vi "Main.vi"(11 "Module Admin":refnum<class "Delacor_lib_QMH_Module Admin.lvclass">) -> ()   [LabVIEW 2020, in "DataBase.lvlib"]
doc: "This template is based off of the Queued Message Handler design pattern and the Queued Message Handler project template that ships with LabVIEW.\n\nThe main difference is that the queue is private to this module and communication between modules is performed via Broadcast and Request events.\n\nRequest events are wrapped in public API methods and are handled in the Event Handling Loop (EHL) of this VI. Any module can register for Broadcast events sent by this module. The EHL generates messages based on user interface actions.\n\nThe Message Handling Loop (MHL) processes messages generated by the EHL, or by other messages. The messages are string values, so new messages can be added easily to the Message Cases case structure in the MHL. Each message cluster can also provide an optional value for Message Data, which is a variant that can be converted to whatever message-specific data is required.\n_____\nBased on Delacor QMH Project Template 5.0.0.82."
uses:
  DataBase.lvlib
  <vilib>/Delacor/Delacor QMH/Libraries/Module Admin_class/Delacor_lib_QMH_Module Admin.lvclass
  Module Data--cluster.ctl
  Acquisition/SignalConfig--cluster.ctl
  Stop Argument--cluster.ctl
  <vilib>/Delacor/Delacor QMH/Libraries/Message Queue_class/Delacor_lib_QMH_Message Queue.lvclass/Delacor_lib_QMH_Message Queue.ctl
  <vilib>/Delacor/Delacor QMH/Libraries/Module Admin_class/Delacor_lib_QMH_Module Admin.lvclass/Delacor_lib_QMH_Module Admin.ctl
  Fetch Data Argument--cluster.ctl
  Fetch Data (Reply Payload)--cluster.ctl
  Save Signal Config Argument--cluster.ctl
  Read Config From DB Argument--cluster.ctl
  Read Config From DB (Reply Payload)--cluster.ctl
  <vilib>/Delacor/Delacor QMH/Libraries/Message Queue_class/Delacor_lib_QMH_Enqueue Message (Single).vi
  <vilib>/Delacor/Delacor QMH/Libraries/Module Admin_class/Delacor_lib_QMH_Get External Launch.vi
  <vilib>/Utility/error.llb/Error Cluster From Error Code.vi
  <vilib>/ErrorRing/Error Ring.xnode
  <vilib>/Delacor/Delacor QMH/Libraries/Message Queue_class/Delacor_lib_QMH_Message Queue.lvclass
panel:
  out "error out":errorcluster
  out "Status":string
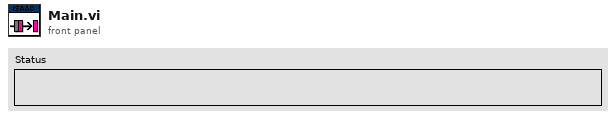
[diagram p1: front panel]
types:
  T1 = typedef "DataBase.lvlib/Request Events--cluster.ctl" = cluster{"Stop Module":refnum<user-event>, "Show Panel":refnum<user-event>, "Hide Panel":refnum<user-event>, "Get Module Execution Status":refnum<user-event>, "Show Diagram":refnum<user-event>, "Fetch Data":refnum<user-event>, "Save config":refnum<user-event>, "Save Signal Config":refnum<user-event>, "Read Config From DB":refnum<user-event>}
  T2 = typedef "DataBase.lvlib/Module Data--cluster.ctl" = cluster{"Status":string, "SignalConfig":T3}
  T3 = typedef "SignalConfig--cluster.ctl" = cluster{"VPP":i32, "Frecuency":dbl, "Offset":dbl, "signal type":enum16{"Sine Wave", "Triangle Wave", "Square Wave", "Sawtooth Wave"}}
  T4 = enum32{"invalid lock state", "Not Locked", "Locked (No Password)", "Password-protected"}
  T5 = typedef "DataBase.lvlib/Stop Argument--cluster.ctl" = cluster{"Origin":string, "Exit via Stop Module Req?":bool, "Wait for Module to stop?":bool}
  T6 = typedef "DataBase.lvlib/Fetch Data Argument--cluster.ctl" = cluster{"End Time":timestamp, "Start Time":timestamp, "Data Results":refnum<vi>, "Wait Notifier":refnum<notifier>, "wait for reply":bool}
  T7 = typedef "DataBase.lvlib/Save Signal Config Argument--cluster.ctl" = cluster{"SignalConfig":T3}
  T8 = typedef "DataBase.lvlib/Read Config From DB Argument--cluster.ctl" = cluster{"Wait Notifier":refnum<notifier>, "wait for reply":bool}
  T9 = enum32{"Invalid", "Standard", "Closed", "Hidden", "Minimized", "Maximized"}
  T10 = typedef "DataBase.lvlib/Fetch Data (Reply Payload)--cluster.ctl" = cluster{"Reply Payload":cluster{"Data":string[][], "Columns":string[], "FetchFrecuencyData_error":errorcluster}}
  T11 = typedef "DataBase.lvlib/Read Config From DB (Reply Payload)--cluster.ctl" = cluster{"SignalConfig":T3, "Read Config From DB_error":errorcluster}
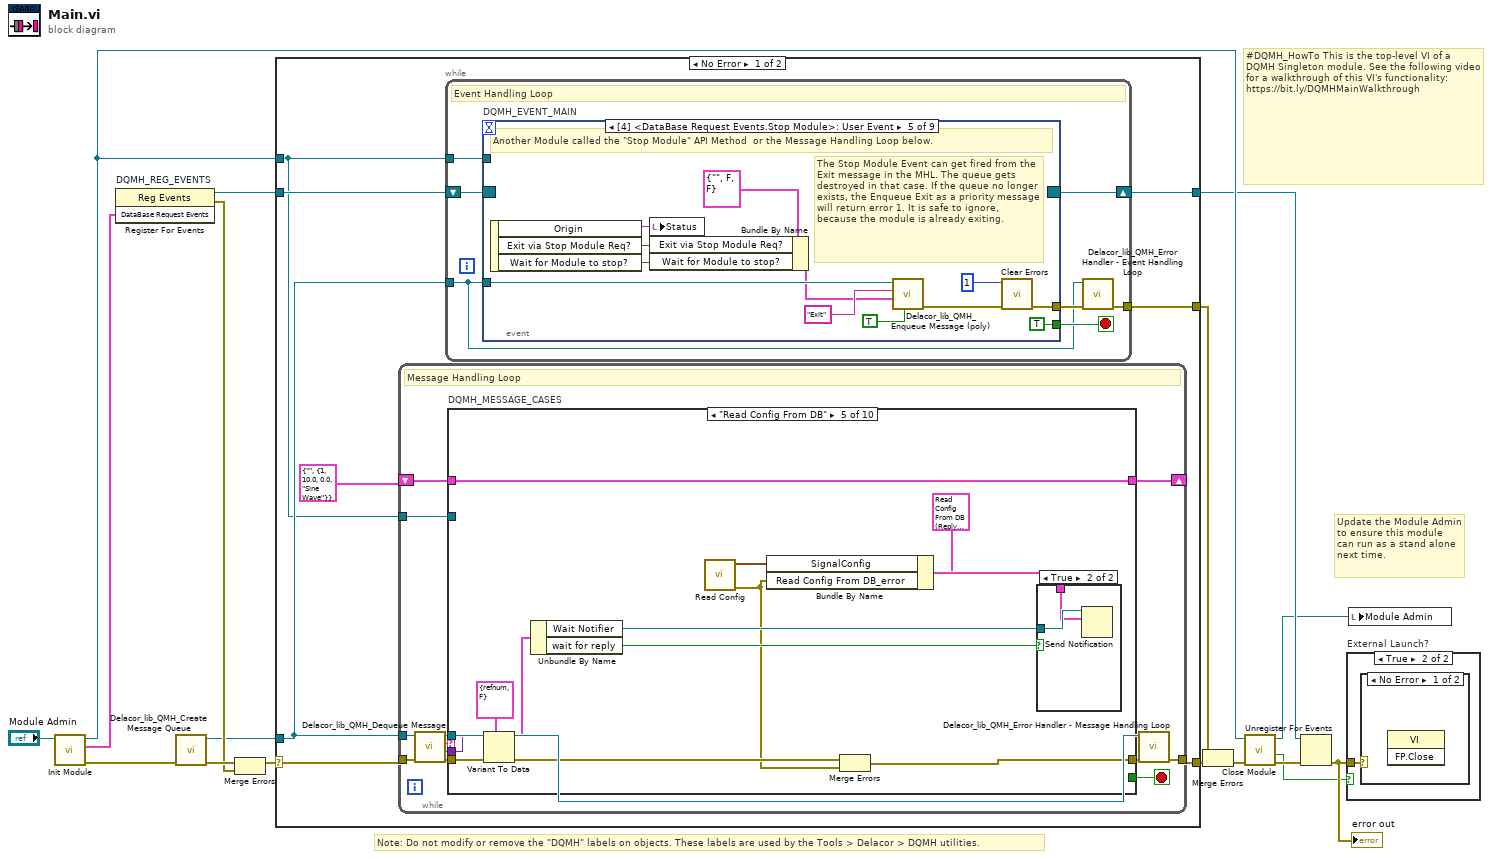
[diagram p0: block diagram]
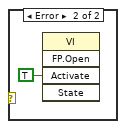
[diagram p3: hidden frame]
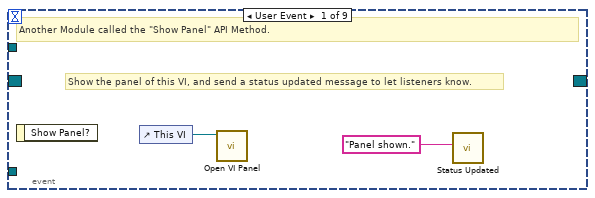
[diagram p4: hidden frame]
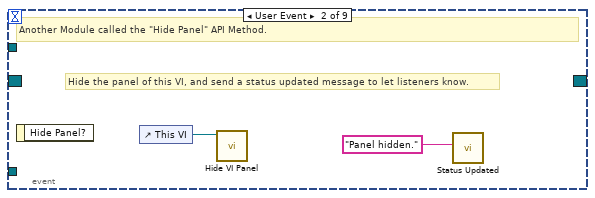
[diagram p5: hidden frame]
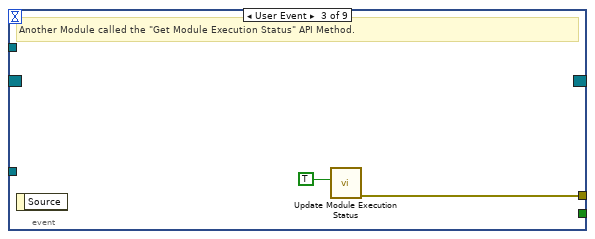
[diagram p6: hidden frame]
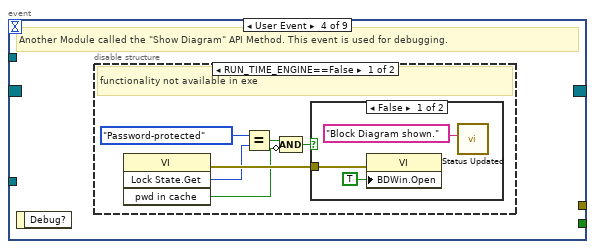
[diagram p7: hidden frame]
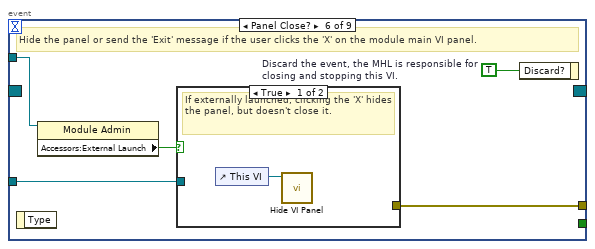
[diagram p10: hidden frame]
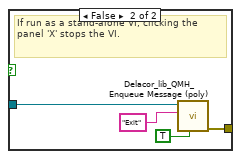
[diagram p11: hidden frame]
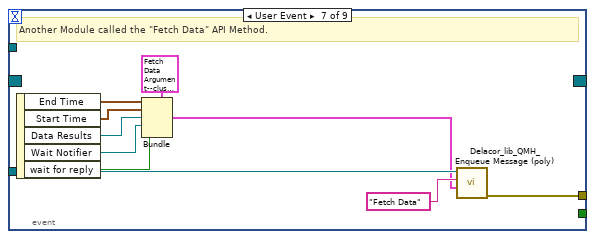
[diagram p12: hidden frame]
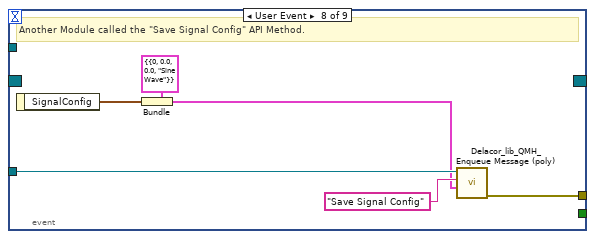
[diagram p13: hidden frame]
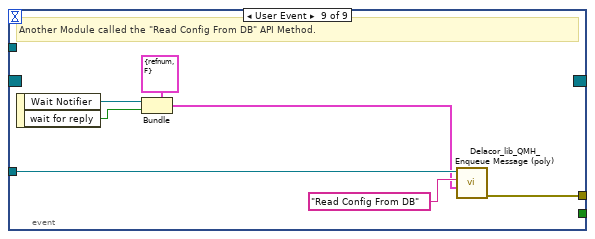
[diagram p14: hidden frame]
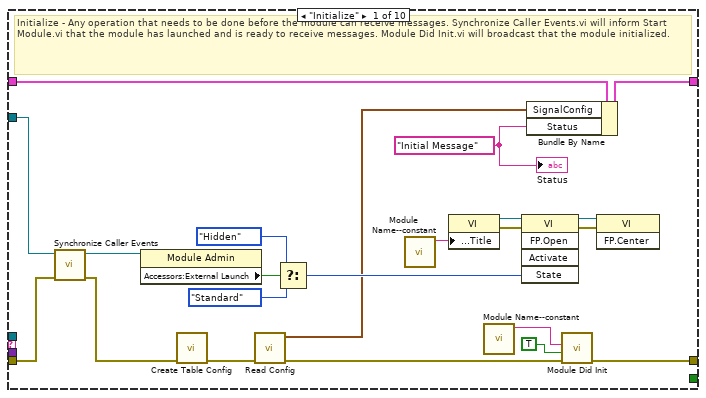
[diagram p15: hidden frame]
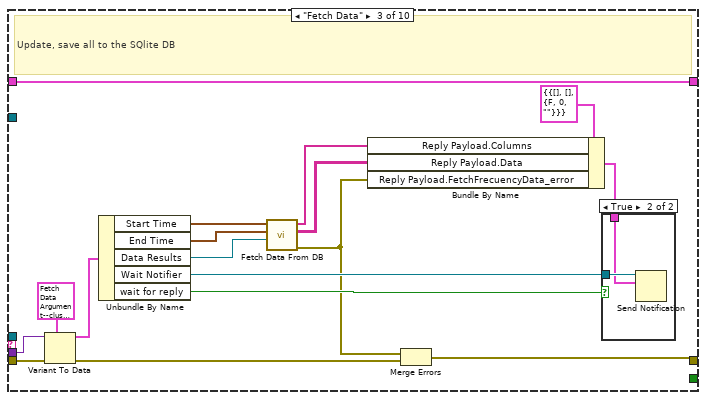
[diagram p17: hidden frame]
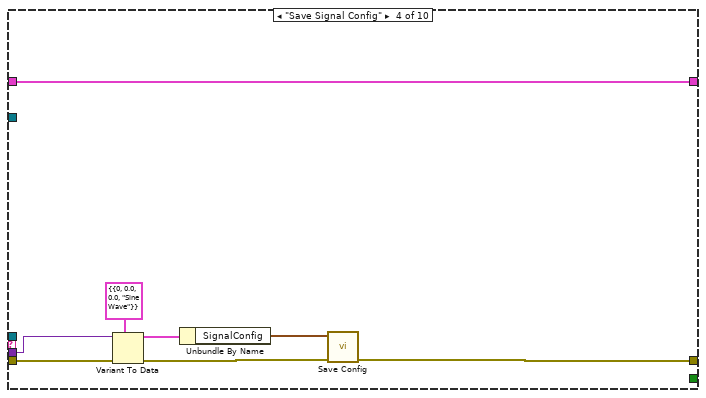
[diagram p19: hidden frame]
diagram:
  # "#DQMH_HowTo This is the top-level VI of a DQMH Singleton module. See the following video for a walkthrough of this VI's functionality: https://bit.ly/DQMHMainWalkthrough"
  # "Note: Do not modify or remove the \"DQMH\" labels on objects. These labels are used by the Tools > Delacor > DQMH utilities."
  # "Update the Module Admin to ensure this module can run as a stand alone next time."
  n1 = call "Init Module.vi"("Singleton Module Admin in"="Module Admin") -> ("error out"=w16:errorcluster, "DataBase Request Events"=w5:T1, "Singleton Module Admin out"=w8:refnum<class "Delacor_lib_QMH_Module Admin.lvclass">)  [unwired: 8 in]
  n2 = register-events "DQMH_REG_EVENTS"(w5) -> (reference out=w6:refnum<event-registration>, error out=w9:errorcluster)  [unwired: 2 in]
  n3 = call <vilib>:"Delacor_lib_QMH_Create Message Queue.vi"("error in"=w16) -> ("error out"=w11:errorcluster, "Message Queue"=w4:refnum<class "Delacor_lib_QMH_Message Queue.lvclass">)  [unwired: 9 in]
  n4 = Merge Errors(w11, w9) -> (w10:errorcluster)
  n5 = case shown="No Error" w10 {
    selector: w10 -> [w23 w223]
    tunnel: [w25 w222] -> w17
    tunnel: [w22 w228] -> w7
    tunnel: w6 -> [w20 w228]
    tunnel: w4 -> [w19 w221]
    tunnel: [w24 _] -> w14
    tunnel: w8 -> [w18 w224]
    frame No Error {
      n6 = while {
        tunnel: w19 -> [w95]
        shift-right: [w99] -> _
        shift-left: T2 {"Status"="", "SignalConfig"={"VPP"=1, "Frecuency"=10.0, "Offset"=0.0, "signal type"=enum."Sine Wave"}} ("Data Cluster") -> [w100]
        tunnel: w23 -> [w103]
        tunnel: [w101] -> w25
        tunnel: w18 -> [w93]
        stop <- w98 stop-if-true
        # "Message Handling Loop"
        n7 = call-dynamic "Delacor_lib_QMH_Dequeue Message.vi"("error in"=w103, "Message Queue in"=w95) -> ("error out"=w102:errorcluster, "Message Data"=w96:variant, "Message"=w97:string, "Message Queue out"=w94:refnum<class "Delacor_lib_QMH_Message Queue.lvclass">)  [unwired: 6 in]
        n8 = case "DQMH_MESSAGE_CASES" shown="\"Read Config From DB\"" w97 {
          selector: w97 -> [_ _ _ _ _ _ _ _ _ w208]
          tunnel: w94 -> [_ _ _ _ _ _ _ w178 w200 _]
          tunnel: w102 -> [w124 w128 w145 w155 w168 w173 w175 w185 w206 w210]
          tunnel: [w123 w128 w135 w148 w158 w172 w175 w181 w203 w211] -> w104
          tunnel: w100 -> [w114 w127 w144 w154 w167 w171 w174 w180 w199 w209]
          tunnel: [w113 w127 w144 w154 w167 w171 w174 w180 w199 w209] -> w99
          tunnel: [_ _ _ _ _ _ _ _ w198 _] -> w98
          tunnel: w96 -> [_ _ w142 w153 w165 _ _ w179 w197 _]
          tunnel: w93 -> [w115 _ _ _ _ _ _ w177 w192 _]
          frame "Initialize" {
            w106 = "Initial Message" ("Initial Message")
            # "Initialize - Any operation that needs to be done before the module can receive messages. Synchronize Caller Events.vi will inform Start Module.vi that the module has launched and is ready to receive messages. Module Did Init.vi will broadcast that the module initialized."
            n9 = call "Synchronize Caller Events.vi"("error in (no error)"=w124, "Singleton Module Admin in"=w115) -> ("error out"=w109:errorcluster, "Singleton Module Admin out"=w110:refnum<class "Delacor_lib_QMH_Module Admin.lvclass">)  [unwired: 8 in]
            n10 = property class="Module Admin"(reference=w110) -> ("Accessors:External Launch"=w119:bool)  [unwired: 1 in, 2 out]
            n11 = call "Create Table Config.vi"("error in (no error)"=w109) -> ("error out"=w108:errorcluster)  [unwired: 10 in]
            n12 = call "Read Config.vi"("error in (no error)"=w108) -> ("error out"=w107:errorcluster, "SignalConfig"=w105:T3)  [unwired: 9 in]
            n13 = Select(t=T9."Hidden" ("State"), s=w119, f=T9."Standard" ("State")) -> (s? t:f=w116:T9)
            n14 = call "Module Name--constant.vi"() -> ("Module Name"=w122:string)  [unwired: 11 in]
            n15 = property class="VI"("Front Panel.Title"=w122) -> (reference out=w121:refnum<vi>, error out=w126:errorcluster)  [unwired: 2 in]
            n16 = call "Module Name--constant.vi"() -> ("Module Name"=w111:string)  [unwired: 11 in]
            n17 = invoke class="VI" method="FP.Open"(reference=w121, error in=w126, "State"=w116) -> (reference out=w120:refnum<vi>, error out=w125:errorcluster)  [unwired: 2 in, 3 out]
            n18 = Bundle By Name(cluster=w114, "SignalConfig"=w105, "Status"=w106) -> (w113:T2)
            n19 = call "Module Did Init.vi"("error in (no error)"=w107, "Initialized?"=TRUE, "Origin"=w111) -> ("error out"=w123:errorcluster)  [unwired: 8 in]
            n20 = invoke class="VI" method="FP.Center"(reference=w120, error in=w125) -> ()  [unwired: 1 in, 3 out]
            "Status" <- w106
          }
          frame "--- Module Specific ---" {
            # "Separator -- The following cases handle messages specific to this Module."
          }
          frame "Fetch Data" {
            # "Update, save all to the SQlite DB"
            n21 = Variant To Data(error in=w145, type=T6 {"End Time"=timestamp(0 s since 1904-01-01), "Start Time"=timestamp(0 s since 1904-01-01), "Data Results"=refnum, "Wait Notifier"=refnum, "wait for reply"=FALSE} ("Fetch Data Argument"), Variant=w142) -> (data=w140:T6, error out=w143:errorcluster)
            n22 = Unbundle By Name(w140) -> ("Start Time"=w134:timestamp, "End Time"=w133:timestamp, "Data Results"=w132:refnum<vi>, "Wait Notifier"=w139:refnum<notifier>, "wait for reply"=w138:bool)
            n23 = call "Fetch Data From DB.vi"("Multicolumn Listbox 2"=w132, "End Time"=w133, "Start Time"=w134) -> ("error out 2"=w129:errorcluster, "Result Set"=w130:string[][], "Column Names"=w131:string[])  [unwired: 6 in]
            n24 = Bundle By Name(cluster=T10 {"Reply Payload"={"Data"=[], "Columns"=[], "FetchFrecuencyData_error"={"status"=FALSE, "code"=0, "source"=""}}} ("Fetch Data (Reply Payload)"), "Reply Payload.Columns"=w131, "Reply Payload.Data"=w130, "Reply Payload.FetchFrecuencyData_error"=w129) -> (w137:T10)
            n25 = Merge Errors(w129, w143) -> (w135:errorcluster)
            n26 = case shown="True" w138 {
              tunnel: w139 -> [_ w147]
              tunnel: w137 -> [_ w146]
              frame False {
              }
              frame True {
                n27 = Send Notification(notification=w146, notifier=w147) -> ()  [unwired: 1 in, 2 out]
              }
            }
          }
          frame "Save Signal Config" {
            n28 = Variant To Data(error in=w155, type=T7 {"SignalConfig"={"VPP"=0, "Frecuency"=0.0, "Offset"=0.0, "signal type"=enum."Sine Wave"}} ("Save Signal Config Argument"), Variant=w153) -> (data=w151:T7, error out=w149:errorcluster)
            n29 = Unbundle By Name(w151) -> ("SignalConfig"=w150:T3)
            n30 = call "Save Config.vi"("error in (no error)"=w149, "SignalConfig"=w150) -> ("error out"=w148:errorcluster)  [unwired: 9 in]
          }
          frame "Read Config From DB" {
            n31 = Variant To Data(error in=w168, type=T8 {"Wait Notifier"=refnum, "wait for reply"=FALSE} ("Read Config From DB Argument"), Variant=w165) -> (data=w163:T8, error out=w166:errorcluster)
            n32 = Unbundle By Name(w163) -> ("Wait Notifier"=w162:refnum<notifier>, "wait for reply"=w161:bool)
            n33 = call "Read Config.vi"() -> ("error out"=w156:errorcluster, "SignalConfig"=w157:T3)  [unwired: 10 in]
            n34 = Bundle By Name(cluster=T11 {"SignalConfig"={"VPP"=0, "Frecuency"=0.0, "Offset"=0.0, "signal type"=enum."Sine Wave"}, "Read Config From DB_error"={"status"=FALSE, "code"=0, "source"=""}} ("Read Config From DB (Reply Payload)"), "SignalConfig"=w157, "Read Config From DB_error"=w156) -> (w160:T11)
            n35 = Merge Errors(w166, w156) -> (w158:errorcluster)
            n36 = case shown="True" w161 {
              tunnel: w162 -> [_ w170]
              tunnel: w160 -> [_ w169]
              frame False {
              }
              frame True {
                n37 = Send Notification(notification=w169, notifier=w170) -> ()  [unwired: 1 in, 2 out]
              }
            }
          }
          frame "---Copy This Frame---" {
            # "Duplicate this frame when creating new messages.  Change this comment in the duplicated frame to describe this message."
            n38 = Merge Errors(w173) -> (w172:errorcluster)
          }
          frame "--- Exit and Error Handling---" {
            # "Separator - The following cases handle errors and exit messages."
          }
          frame "Error" {
            # "#CodeRecommended - If you ever change the name of this \"Error\" message, you'll need to update the name in the Check Loop Error.vi as well."
            # "#CodeRecommended - If the module is running in standalone mode (External Launch = FALSE), this code will pop up an error dialog and call the 'Exit' message if an error occurs. Add more fine-grained error handling here."
            # "Error - Check the error message data and respond accordingly. This message is sent by the \"Error Handler\" VIs at the end of each loop in this application."
            n39 = property class="Module Admin"(reference=w177) -> ("Accessors:External Launch"=w176:bool)  [unwired: 1 in, 2 out]
            n40 = Variant To Data(error in=w185, type=errorcluster {"status"=FALSE, "code"=0, "source"=""} ("error constant"), Variant=w179) -> (data=w186:errorcluster, error out=w183:errorcluster)
            n41 = call "Error Reported.vi"("Error"=w186) -> ()  [unwired: 10 in, 1 out]
            n42 = case shown="False" w176 {
              tunnel: [w191 _] -> w182
              tunnel: w178 -> [w189 _]
              tunnel: w186 -> [w190 _]
              frame False {
                # "If the module is running standalone, then pop up an error dialog and call the \"Exit\" message."
                n43 = call <vilib>:"Simple Error Handler.vi"("error in (no error)"=w190) -> ()  [unwired: 4 in, 5 out]
                n44 = call-poly <vilib>:"Delacor_lib_QMH_Enqueue Message (poly).vi"("Priority Message? (F)"=TRUE, "Message"="Exit", "Message Queue in"=w189) -> ("error out"=w191:errorcluster)  [unwired: 7 in, 1 out]
              }
              frame True {
                # "If the module was launched externally, calling the Error Reported broadcast VI is the only action performed by the \"Error\" message. The module's caller can then process the error appropriately."
              }
            }
            n45 = Merge Errors(w183, w182) -> (w181:errorcluster)
            n46 = local write "error out"(w181) -> ()
          }
          frame "Exit" {
            w196 = 91  # 91: not all Exit messages will have an argument
            w198 = TRUE  # Stop the VI
            # "Release the message queue reference"
            # "#CodeNeeded - Add any required cleanup code here"
            # "Exit - Exit the application."
            n47 = Variant To Data(error in=w206, type=T5 {"Origin"="", "Exit via Stop Module Req?"=FALSE, "Wait for Module to stop?"=FALSE} ("Stop Argument"), Variant=w197) -> (data=w194:T5, error out=w202:errorcluster)
            n48 = call <vilib>:"Clear Errors.vi"("error in (no error)"=w202, "specific error code to clear (0: all)"=w196) -> ("error out"=w205:errorcluster)  [unwired: 4 in, 1 out]
            n49 = control-ref of="This VI"() -> (w193:refnum<vi>)
            n50 = call-dynamic "Delacor_lib_QMH_Release Message Queue.vi"("error in"=w205, "Message Queue"=w200) -> ("error out"=w204:errorcluster)  [unwired: 9 in]
            n51 = call "Handle Exit.vi"("Stop Argument"=w194, "Admin in"=w192, "VI reference"=w193) -> ("error out"=w201:errorcluster)  [unwired: 7 in, 1 out]
            n52 = Merge Errors(w204, w201) -> (w203:errorcluster)
          }
          frame Default {
            # "'Default' case only runs if there is a message that isn't defined in any of the other cases.  Output a programming error."
            n53 = call "Module Name--constant.vi"() -> ("Module Name"=w207:string)  [unwired: 11 in]
            n54 = xnode "Error Ring"("parameter 0"=w208, "parameter 1"=w207) -> ("error out"=w212:errorcluster)
            n55 = Merge Errors(w210, w212) -> (w211:errorcluster)
          }
        }
        n56 = call-dynamic "Delacor_lib_QMH_Error Handler - Message Handling Loop.vi"("error in"=w104, "Message Queue in"=w94) -> ("dup error in"=w101:errorcluster)  [unwired: 8 in, 1 out]
      }
      n57 = while {
        tunnel: w19 -> [w26]
        shift-right: [w29] -> w22
        shift-left: w20 -> [w30]
        tunnel: [w31] -> w24
        tunnel: w18 -> [w27]
        stop <- w28 stop-if-true
        # "Event Handling Loop"
        n58 = event "DQMH_EVENT_MAIN" shown="[4] <DataBase Request Events.Stop Module>: User Event" {
          selector: w30 -> [_ _ _ _ _ _ _ _ _]
          dyn-events: [_ _ _ _ _ _ _ _ _] -> w29
          timeout: _ -> [_ _ _ _ _ _ _ _ _]
          tunnel: [_ _ _ _ TRUE ("Discard?") _ _ _ _] -> w28
          tunnel: w26 -> [_ _ _ _ w55 w62 w79 w85 w92]
          tunnel: [_ _ w38 _ w58 w64 w70 w80 w86] -> w32
          tunnel: w27 -> [_ _ _ _ _ w61 _ _ _]
          event User Event {
            # "Show the panel of this VI, and send a status updated message to let listeners know."
            # "Another Module called the \"Show Panel\" API Method."
            n59 = event-data() -> ()  [unwired: 1 in, 1 out]
            n60 = control-ref of="This VI"() -> (w34:refnum<vi>)
            n61 = call "Open VI Panel.vi"("VI"=w34) -> ()  [unwired: 10 in, 1 out]
            n62 = call "Status Updated.vi"("Status"="Panel shown." ("format string")) -> ()  [unwired: 10 in, 1 out]
          }
          event User Event {
            # "Hide the panel of this VI, and send a status updated message to let listeners know."
            # "Another Module called the \"Hide Panel\" API Method."
            n63 = event-data() -> ()  [unwired: 1 in, 1 out]
            n64 = control-ref of="This VI"() -> (w36:refnum<vi>)
            n65 = call "Hide VI Panel.vi"("VI"=w36) -> ()  [unwired: 10 in, 1 out]
            n66 = call "Status Updated.vi"("Status"="Panel hidden." ("format string")) -> ()  [unwired: 10 in, 1 out]
          }
          event User Event {
            # "Another Module called the \"Get Module Execution Status\" API Method."
            n67 = event-data() -> ()  [unwired: 1 in, 1 out]
            n68 = call "Update Module Execution Status.vi"("Running?"=TRUE) -> ("error out"=w38:errorcluster)  [unwired: 10 in]
          }
          event User Event {
            # "Another Module called the \"Show Diagram\" API Method. This event is used for debugging."
            n69 = event-data() -> ()  [unwired: 1 in, 1 out]
            n70 = disable-structure shown="RUN_TIME_ENGINE==False" {
              frame condition #0 (active) {
                # "functionality not available in exe"
                n71 = invoke class="VI" method="Lock State.Get"() -> (error out=w44:errorcluster, "Get Lock State"=w43:T4, "pwd in cache"=w40:bool)  [unwired: 4 in, 1 out]
                n72 = Equal?(x=T4."Password-protected", y=w43) -> (x = y?=w41:bool)
                n73 = Compound Arithmetic op=AND(w41, invert w40) -> (w39:bool)
                n74 = case shown="False" w39 {
                  tunnel: w44 -> [w47 _]
                  frame False {
                    n75 = property class="VI"(error in=w47, "BDWin.Open"=TRUE ("Block Diagram Window:Open")) -> ()  [unwired: 1 in, 2 out]
                    n76 = call "Status Updated.vi"("Status"="Block Diagram shown." ("format string")) -> ()  [unwired: 10 in, 1 out]
                  }
                  frame True {
                    # "Password-protected VI, and the password is not in the cache. Do not show the diagram."
                  }
                }
              }
              frame condition #1 {
              }
            }
          }
          event User Event {
            # "The Stop Module Event can get fired from the Exit message in the MHL. The queue gets destroyed in that case. If the queue no longer exists, the Enqueue Exit as a priority message will return error 1. It is safe to ignore, because the module is already exiting."
            # "Another Module called the \"Stop Module\" API Method  or the Message Handling Loop below."
            n77 = event-data() -> ("Origin"=w54:string, "Exit via Stop Module Req?"=w50:bool, "Wait for Module to stop?"=w49:bool)  [unwired: 1 in]
            n78 = local write "Status"(w54) -> ()
            n79 = Bundle By Name(cluster=T5 {"Origin"="", "Exit via Stop Module Req?"=FALSE, "Wait for Module to stop?"=FALSE} ("Stop Argument"), "Exit via Stop Module Req?"=w50, "Wait for Module to stop?"=w49) -> (w48:T5)
            n80 = call-poly <vilib>:"Delacor_lib_QMH_Enqueue Message (poly).vi"("Priority Message? (F)"=TRUE, "Message Data"=w48, "Message"="Exit", "Message Queue in"=w55) -> ("error out"=w59:errorcluster)  [unwired: 6 in, 1 out]
            n81 = call <vilib>:"Clear Errors.vi"("error in (no error)"=w59, "specific error code to clear (0: all)"=1) -> ("error out"=w58:errorcluster)  [unwired: 4 in, 1 out]
          }
          event Panel Close? {
            w63 = TRUE  # Discard the event, the MHL is responsible for closing and stopping this VI.
            # "Hide the panel or send the 'Exit' message if the user clicks the 'X' on the module main VI panel."
            n82 = event-data() -> ()  [unwired: 1 in, 1 out]
            n83 = property class="Module Admin"(reference=w61) -> ("Accessors:External Launch"=w60:bool)  [unwired: 1 in, 2 out]
            n84 = case shown="True" w60 {
              tunnel: w62 -> [_ w68]
              tunnel: [_ w69] -> w64
              frame True {
                # "If externally launched, clicking the 'X' hides the panel, but doesn't close it."
                n85 = control-ref of="This VI"() -> (w65:refnum<vi>)
                n86 = call "Hide VI Panel.vi"("VI"=w65) -> ()  [unwired: 10 in, 1 out]
              }
              frame False {
                # "If run as a stand-alone VI, clicking the panel 'X' stops the VI."
                n87 = call-poly <vilib>:"Delacor_lib_QMH_Enqueue Message (poly).vi"("Priority Message? (F)"=TRUE, "Message"="Exit", "Message Queue in"=w68) -> ("error out"=w69:errorcluster)  [unwired: 7 in, 1 out]
              }
            }
            n88 = event-data("Discard?"=w63) -> ()  [unwired: 1 in, 1 out]
          }
          event User Event {
            # "Another Module called the \"Fetch Data\" API Method."
            n89 = event-data() -> ("End Time"=w75:timestamp, "Start Time"=w74:timestamp, "Data Results"=w73:refnum<vi>, "Wait Notifier"=w72:refnum<notifier>, "wait for reply"=w71:bool)  [unwired: 1 in]
            n90 = Bundle(cluster=T6 {"End Time"=timestamp(0 s since 1904-01-01), "Start Time"=timestamp(0 s since 1904-01-01), "Data Results"=refnum, "Wait Notifier"=refnum, "wait for reply"=FALSE} ("Fetch Data Argument"), "End Time"=w75, "Start Time"=w74, "Data Results"=w73, "Wait Notifier"=w72, "wait for reply"=w71) -> (w76:T6)
            n91 = call-poly <vilib>:"Delacor_lib_QMH_Enqueue Message (poly).vi"("Message Data"=w76, "Message"="Fetch Data", "Message Queue in"=w79) -> ("error out"=w70:errorcluster)  [unwired: 7 in, 1 out]
          }
          event User Event {
            # "Another Module called the \"Save Signal Config\" API Method."
            n92 = event-data() -> ("SignalConfig"=w81:T3)  [unwired: 1 in]
            n93 = Bundle(cluster=T7 {"SignalConfig"={"VPP"=0, "Frecuency"=0.0, "Offset"=0.0, "signal type"=enum."Sine Wave"}} ("Save Signal Config Argument"), "SignalConfig"=w81) -> (w82:T7)
            n94 = call-poly <vilib>:"Delacor_lib_QMH_Enqueue Message (poly).vi"("Message Data"=w82, "Message"="Save Signal Config", "Message Queue in"=w85) -> ("error out"=w80:errorcluster)  [unwired: 7 in, 1 out]
          }
          event User Event {
            # "Another Module called the \"Read Config From DB\" API Method."
            n95 = event-data() -> ("Wait Notifier"=w88:refnum<notifier>, "wait for reply"=w87:bool)  [unwired: 1 in]
            n96 = Bundle(cluster=T8 {"Wait Notifier"=refnum, "wait for reply"=FALSE} ("Read Config From DB Argument"), "Wait Notifier"=w88, "wait for reply"=w87) -> (w89:T8)
            n97 = call-poly <vilib>:"Delacor_lib_QMH_Enqueue Message (poly).vi"("Message Data"=w89, "Message"="Read Config From DB", "Message Queue in"=w92) -> ("error out"=w86:errorcluster)  [unwired: 7 in, 1 out]
          }
        }
        n98 = call-dynamic "Delacor_lib_QMH_Error Handler - Event Handling Loop.vi"("error in"=w32, "Message Queue in"=w26) -> ("dup error in"=w31:errorcluster)  [unwired: 8 in, 1 out]
      }
    }
    frame Error {
      # "Synchronize Caller Events.vi will inform Start Module.vi that the module has launched and will let the code calling Start Module.vi register for broadcasts and would permit the caller receive the broadcast that an error occurred at launch time."
      n99 = call-dynamic "Delacor_lib_QMH_Release Message Queue.vi"("error in"=w223, "Message Queue"=w221) -> ("error out"=w222:errorcluster)  [unwired: 9 in]
      n100 = call "Synchronize Caller Events.vi"("Singleton Module Admin in"=w224) -> ("error out"=w229:errorcluster)  [unwired: 9 in, 1 out]
      n101 = call "Module Name--constant.vi"() -> ("Module Name"=w227:string)  [unwired: 11 in]
      n102 = Format Into String(format string="An error occurred during initialization. %s is no longer running.", w227) -> (resulting string=w225:string)  [unwired: 2 in, 1 out]
      n103 = Merge Errors(w222, w229) -> (w230:errorcluster)
      n104 = call "Error Reported.vi"("Additional Information"=w225, "Error"=w230) -> ()  [unwired: 9 in, 1 out]
    }
  }
  n105 = Merge Errors(w14, w17) -> (w13:errorcluster)
  n106 = call "Close Module.vi"("error in (no error)"=w13, "Module Admin in"=w8) -> ("error out"=w15:errorcluster, "External Launch"=w1:bool, "Module Admin out"=w2:refnum<class "Delacor_lib_QMH_Module Admin.lvclass">)  [unwired: 7 in]
  n107 = Unregister For Events(event registration refnum=w7, error in=w15) -> (error out=w12:errorcluster)
  "error out" <- w12
  n108 = case "External Launch?" shown="True" w1 {
    tunnel: w12 -> [_ w231]
    frame False {
    }
    frame True {
      n109 = case shown="No Error" w231 {
        frame No Error {
          n110 = invoke class="VI" method="FP.Close"() -> ()  [unwired: 3 in, 3 out]
        }
        frame Error {
          n111 = invoke class="VI" method="FP.Open"("Activate"=TRUE ("Activate?")) -> ()  [unwired: 4 in, 5 out]
        }
      }
    }
  }
  n112 = local write "Module Admin"(w2) -> ()
